vi "BeamGage Chart.vi"() -> ()   [LabVIEW 2009]
uses:
  C:/Program Files/Spiricon/BeamGage Professional/Spiricon.BeamGage.Automation.dll
  C:/Program Files/Spiricon/BeamGage Professional/Spiricon.Automation.dll
panel:
  out "Status":i32(ring) items=["NOT_SUPPORTED", "FAILED", "CALIBRATING", "READY", "BEAM_DETECTED"]
  out "2D Intensity Graph":dbl[][](graph)
  out "1D Profile - Peak Location Y - Waveform Graph":dbl[](graph)
  out "Height":dbl
  out "Width":dbl
  out "Peak Loc Y":dbl
  out "Peak Loc X":dbl
  in  "START_STOP":bool
  in  "ULTRACAL":bool
  out "Total and Peak Power - Waveform Chart":cluster{"Total":dbl, "Peak":dbl}(graph)
  in  "STOP SERVER":bool
  # "Block laser beam and \nclick Ultracal to calibrate"
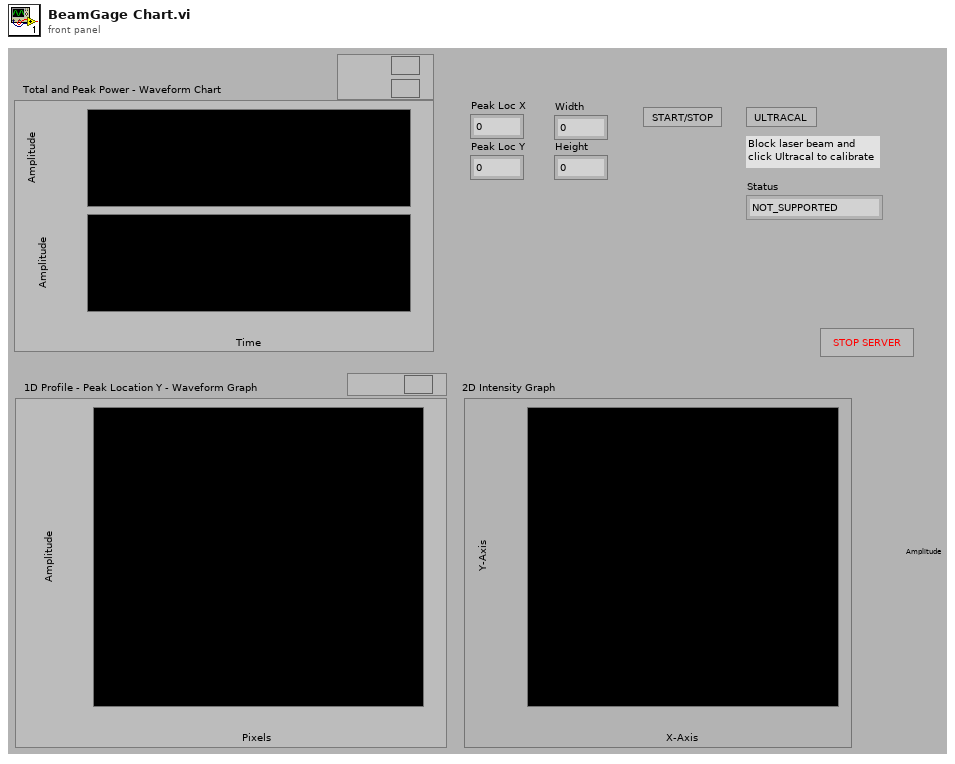
[diagram p1: front panel]
types:
  T1 = cluster{"Total":dbl, "Peak":dbl, "Peak X":dbl, "Peak Y":dbl, "Width":dbl, "Height":dbl, "DoubleData":dbl[], "Scale Multiplier":dbl}
  T2 = cluster{"notifier out":refnum<notifier>, "new reference":refnum<k24>}
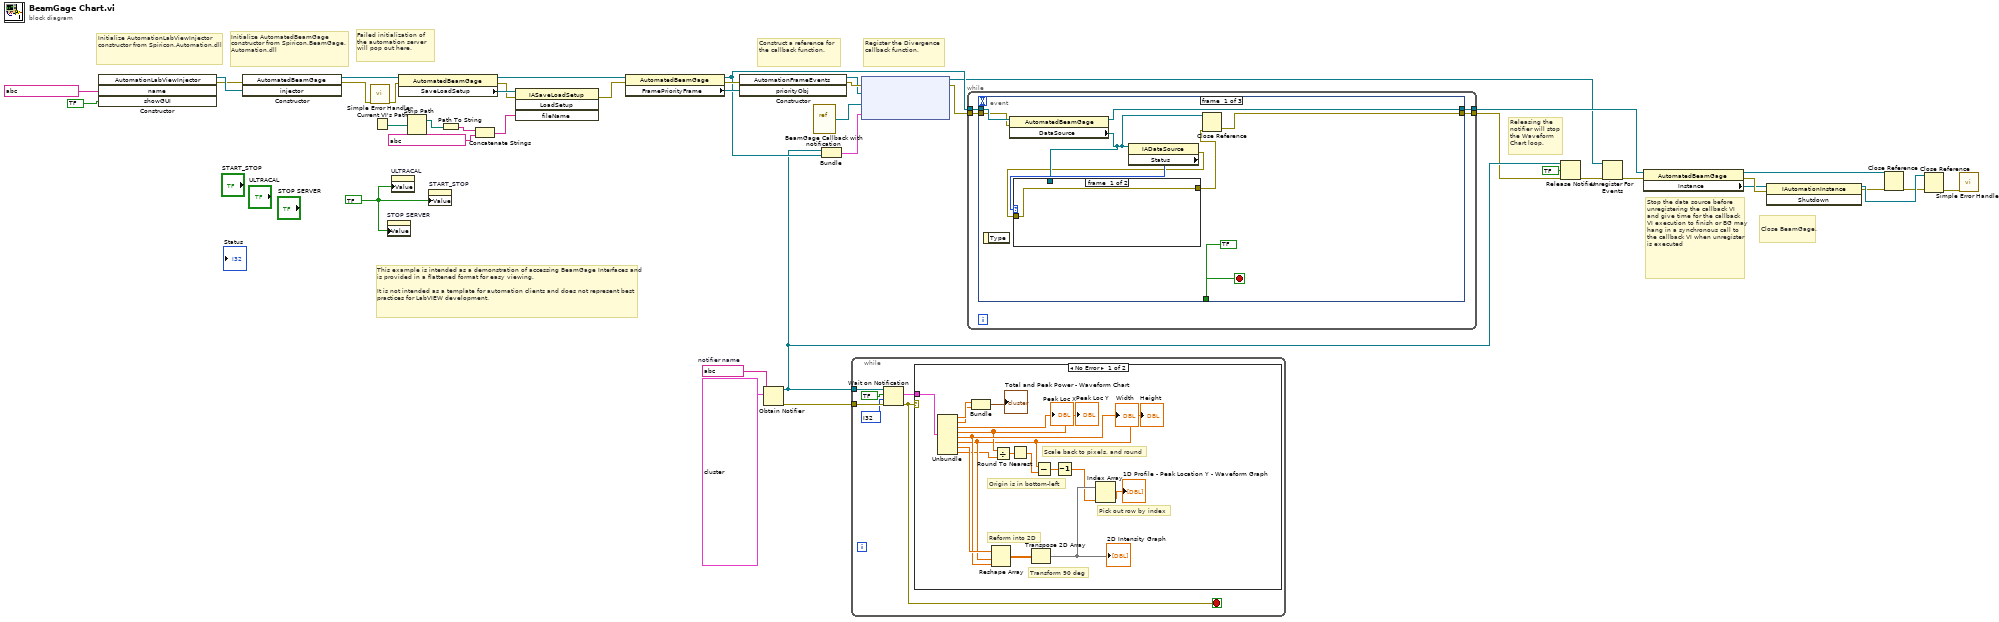
[diagram p0: block diagram]
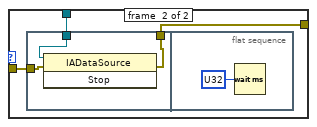
[diagram p2: hidden frame]
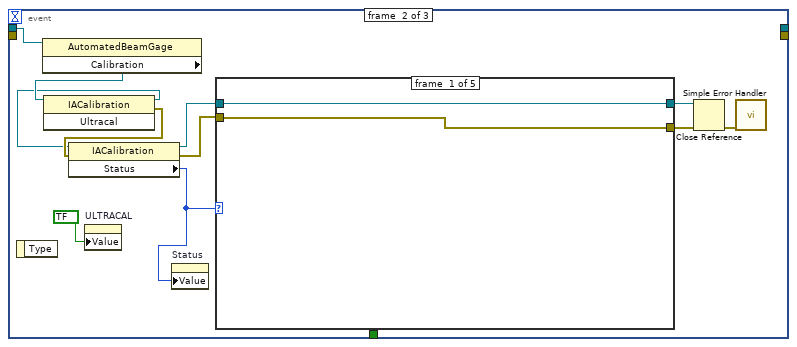
[diagram p3: hidden frame]
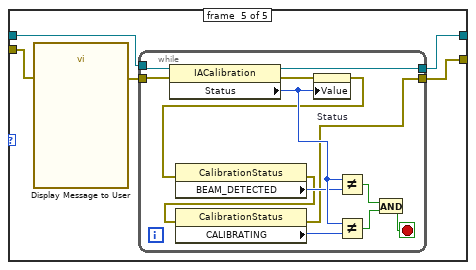
[diagram p7: hidden frame]
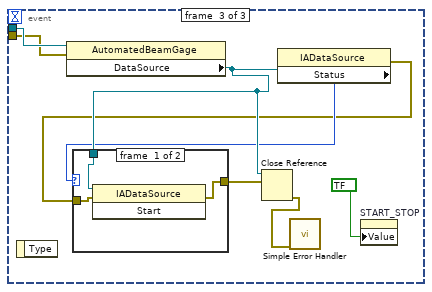
[diagram p8: hidden frame]
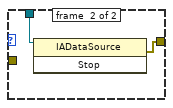
[diagram p9: hidden frame]
diagram:
  w39 = bool ? ("stop")
  w42 = string ?  # notifier name
  # "Initialize AutomationLabViewInjector constructor from Spiricon.Automation.dll"
  # "Failed initialization of the automation server will pop out here."
  # "This example is intended as a demonstration of accessing BeamGage Interfaces and is provided in a flattened format for easy viewing.\n\nIt is not intended as a template for automation clients and does not represent best practices for LabVIEW development."
  # "Stop the data source before unregistering the callback VI  and give time for the callback VI execution to finish or BG may hang in a synchronous call to the callback VI when unregister is executed"
  # "Releasing the notifier will stop the Waveform Chart loop."
  # "Close BeamGage."
  # "Initialize AutomatedBeamGage constructor from Spiricon.BeamGage.Automation.dll"
  # "Register the Divergence callback function."
  # "Construct a reference for the callback function."
  n1 = constructor class="AutomationLabViewInjector"("name"=string ? ("Name"), "showGUI"=bool ? ("LaunchUI")) -> (reference out=w4:refnum<k24>, error out=w1:errorcluster)  [unwired: 3 in, 3 out]
  n2 = constructor class="AutomatedBeamGage"(error in=w1, "injector"=w4) -> (reference out=w35:refnum<k24>, error out=w6:errorcluster)  [unwired: 2 in, 2 out]
  n3 = call <vilib>:"Simple Error Handler.vi"("error in (no error)"=w6) -> ("error out"=w5:errorcluster)  [unwired: 4 in, 4 out]
  n4 = Current VI's Path() -> (path=w28:path)
  n5 = property on="STOP SERVER" class="Bool (strict)"("Value"=w39) -> ()  [unwired: 2 in, 2 out]
  n6 = property on="ULTRACAL" class="Bool (strict)"("Value"=w39) -> ()  [unwired: 2 in, 2 out]
  n7 = property class="AutomatedBeamGage"(reference=w35, error in=w5) -> (reference out=w31:refnum<k24>, error out=w33:errorcluster, "SaveLoadSetup"=w34:refnum<k24>)
  n8 = Strip Path(path=w28) -> (stripped path=w27:path)  [unwired: 1 out]
  n9 = property on="START_STOP" class="Bool (strict)"("Value"=w39) -> ()  [unwired: 2 in, 2 out]
  n10 = Path To String(path=w27) -> (string=w30:string)
  n11 = Concatenate Strings(w30, string ? ("string")) -> (w26:string)
  n12 = invoke class="IASaveLoadSetup" method="LoadSetup"(reference=w34, error in=w33, "fileName"=w26) -> (error out=w32:errorcluster)  [unwired: 1 in, 3 out]
  n13 = property class="AutomatedBeamGage"(reference=w31, error in=w32) -> (reference out=w36:refnum<k24>, error out=w37:errorcluster, "FramePriorityFrame"=w38:refnum<k24>)
  n14 = constructor class="AutomationFrameEvents"(error in=w37, "priorityObj"=w38) -> (reference out=w24:refnum<k24>, error out=w25:errorcluster)  [unwired: 2 in, 2 out]
  n15 = Obtain Notifier(name (unnamed)=w42, notification data type=T1 ?) -> (notifier out=w9:refnum<notifier>, error out=w40:errorcluster)  [unwired: 2 in, 1 out]
  n16 = vi-ref "BeamGage Callback with notification.vi"() -> ("vi reference"=w21:refnum<vi>)
  n17 = Bundle("notifier out"=w9, "new reference"=w36) -> (w22:T2)  [unwired: 1 in]
  n18 = while {
    tunnel: w9 -> [w48]
    tunnel: w40 -> [w46]
    stop <- w44 stop-if-true
    n19 = Wait on Notification(notifier=w48, ignore previous (F)=bool ?, timeout in ms (-1)=i32 ?, error in (no error)=w46) -> (notification=w47:T1, error out=w44:errorcluster)  [unwired: 2 out]
    n20 = case shown="No Error" w44 {
      tunnel: w47 -> [w65 _]
      frame #0 {
        # "Transform 90 deg"
        # "Scale back to pixels, and round"
        # "Pick out row by index"
        # "Reform into 2D"
        # "Origin is in bottom-left"
        n21 = Unbundle(w65) -> ("Total"=w64:dbl, "Peak"=w63:dbl, "Peak X"=→"Peak Loc X":dbl, "Peak Y"=w54:dbl, "Width"=w56:dbl, "Height"=w52:dbl, "DoubleData"=w59:dbl[], "Scale Multiplier"=w49:dbl)
        "Peak Loc Y" <- w54
        "Width" <- w56
        "Height" <- w52
        n22 = Bundle("Total"=w64, "Peak"=w63) -> (→"Total and Peak Power - Waveform Chart":cluster{"Total":dbl, "Peak":dbl})  [unwired: 1 in]
        n23 = Reshape Array(w59, w52, w56) -> (w58:dbl[][])
        n24 = Divide(x=w54, y=w49) -> (x/y=w55:dbl)
        n25 = Round To Nearest(number=w55) -> (nearest integer value=w51:dbl)
        n26 = Transpose 2D Array(2D array=w58) -> (transposed array=w57:dbl[][])
        "2D Intensity Graph" <- w57
        n27 = Subtract(x=w52, y=w51) -> (x-y=w53:dbl)
        n28 = Decrement(x=w53) -> (x-1=w50:dbl)
        n29 = Index Array(array=w57, index (col)=w50) -> (element=→"1D Profile - Peak Location Y - Waveform Graph":dbl[])  [unwired: 1 in]
      }
      frame #1 {
        # "Don't update chart when an error occurs."
      }
    }
  }
  n30 = node(w25, w24, w21, w22) -> (w10:refnum<k27>, w23:errorcluster)  [unwired: 1 in]
  n31 = while {
    tunnel: [w70] -> w11
    tunnel: w36 -> [w69]
    tunnel: w23 -> [w67]
    tunnel: [w66] -> w8
    stop <- w68 stop-if-true
    n32 = event shown="[1] \"ULTRACAL\": Mouse Down" {
      selector: _ -> [_ _ _]
      dyn-events: _ -> [_ _ _]
      timeout: _ -> [_ _ _]
      tunnel: w69 -> [w77 w97 w129]
      tunnel: [w76 _ _] -> w70
      tunnel: [bool ? ("stop") _ _] -> w68
      tunnel: w67 -> [w75 _ w128]
      tunnel: [w78 _ _] -> w66
      event #0 {
        n33 = event-data() -> ()  [unwired: 1 in, 1 out]
        n34 = property class="AutomatedBeamGage"(reference=w77, error in=w75) -> (reference out=w76:refnum<k24>, "DataSource"=w73:refnum<k24>)  [unwired: 1 out]
        n35 = property class="IADataSource"(reference=w73) -> (error out=w71:errorcluster, "Status"=w74:i32)  [unwired: 1 in, 1 out]
        n36 = case shown="1" w74 {
          tunnel: w73 -> [_ w83]
          tunnel: [w80 w82] -> w72
          tunnel: w71 -> [w80 w81]
          frame #0 {
          }
          frame #1 {
            n37 = flat-sequence {
              tunnel: w83 -> [w86]
              tunnel: [w85] -> w82
              tunnel: w81 -> [w84]
              frame #0 {
                n38 = invoke class="IADataSource" method="Stop"(reference=w86, error in=w84) -> (error out=w85:errorcluster)  [unwired: 1 in, 2 out]
              }
              frame #1 {
                n39 = Wait (ms)(milliseconds to wait=u32 ?) -> ()  [unwired: 1 out]
              }
            }
          }
        }
        n40 = Close Reference(reference=w73, error in (no error)=w72) -> (error out=w78:errorcluster)
      }
      event #1 {
        n41 = event-data() -> ()  [unwired: 1 in, 1 out]
        n42 = property class="AutomatedBeamGage"(reference=w97) -> ("Calibration"=w96:refnum<k24>)  [unwired: 1 in, 2 out]
        n43 = invoke class="IACalibration" method="Ultracal"(reference=w96) -> (reference out=w94:refnum<k24>, error out=w95:errorcluster)  [unwired: 2 in, 1 out]
        n44 = property class="IACalibration"(reference=w94, error in=w95) -> (reference out=w93:refnum<k24>, error out=w92:errorcluster, "Status"=w91:i32)
        n45 = property on="ULTRACAL" class="Bool (strict)"("Value"=bool ? ("stop")) -> ()  [unwired: 2 in, 2 out]
        n46 = property on="Status" class="Ring (strict)"("Value"=w91) -> ()  [unwired: 2 in, 2 out]
        n47 = case shown="4" w91 {
          tunnel: [w99 w101 w103 w105 w107] -> w88
          tunnel: [w100 w102 w104 w106 w109] -> w89
          tunnel: w93 -> [w100 w102 w104 w106 w110]
          tunnel: w92 -> [w99 w101 w103 w105 w111]
          frame #0 {
          }
          frame #1 {
          }
          frame #2 {
          }
          frame #3 {
          }
          frame #4 {
            n48 = call "Display Message to User"("error in (no error)"=w111) -> ("error out"=w108:errorcluster)  [unwired: 9 in, 1 out]
            n49 = while {
              tunnel: w110 -> [w124]
              tunnel: [w123] -> w109
              tunnel: w108 -> [w122]
              tunnel: [w112] -> w107
              stop <- w120 stop-if-true
              n50 = property class="IACalibration"(reference=w124, error in=w122) -> (reference out=w123:refnum<k24>, error out=w121:errorcluster, "Status"=w117:i32)
              n51 = property on="Status" class="Ring (strict)"(error in=w121, "Value"=w117) -> (error out=w116:errorcluster)  [unwired: 1 in, 1 out]
              n52 = property class="CalibrationStatus"(error in=w116) -> (error out=w113:errorcluster, "BEAM_DETECTED"=w115:i32)  [unwired: 1 in, 1 out]
              n53 = property class="CalibrationStatus"(error in=w113) -> (error out=w112:errorcluster, "CALIBRATING"=w114:i32)  [unwired: 1 in, 1 out]
              n54 = Not Equal?(x=w117, y=w115) -> (x != y?=w118:bool)
              n55 = Not Equal?(x=w117, y=w114) -> (x != y?=w119:bool)
              n56 = And(x=w118, y=w119) -> (x .and. y?=w120:bool)
            }
          }
        }
        n57 = Close Reference(reference=w89, error in (no error)=w88) -> (error out=w90:errorcluster)
        n58 = call <vilib>:"Simple Error Handler.vi"("error in (no error)"=w90) -> ()  [unwired: 4 in, 5 out]
      }
      event #2 {
        n59 = event-data() -> ()  [unwired: 1 in, 1 out]
        n60 = property class="AutomatedBeamGage"(reference=w129, error in=w128) -> ("DataSource"=w127:refnum<k24>)  [unwired: 2 out]
        n61 = property class="IADataSource"(reference=w127) -> (error out=w125:errorcluster, "Status"=w126:i32)  [unwired: 1 in, 1 out]
        n62 = case shown="1" w126 {
          tunnel: [w133 w137] -> w131
          tunnel: w127 -> [w135 w136]
          tunnel: w125 -> [w134 _]
          frame #0 {
            n63 = invoke class="IADataSource" method="Start"(reference=w135, error in=w134) -> (error out=w133:errorcluster)  [unwired: 1 in, 2 out]
          }
          frame #1 {
            n64 = invoke class="IADataSource" method="Stop"(reference=w136) -> (error out=w137:errorcluster)  [unwired: 2 in, 2 out]
          }
        }
        n65 = Close Reference(reference=w127, error in (no error)=w131) -> (error out=w130:errorcluster)
        n66 = call <vilib>:"Simple Error Handler.vi"("error in (no error)"=w130) -> ()  [unwired: 4 in, 5 out]
        n67 = property on="START_STOP" class="Bool (strict)"("Value"=bool ? ("stop")) -> ()  [unwired: 2 in, 2 out]
      }
    }
  }
  n68 = Release Notifier(notifier=w9, force destroy? (F)=bool ?, error in (no error)=w8) -> (error out=w12:errorcluster)  [unwired: 2 out]
  n69 = Unregister For Events(event registration refnum=w10, error in=w12) -> (error out=w16:errorcluster)
  n70 = property class="AutomatedBeamGage"(reference=w11, error in=w16) -> (reference out=w15:refnum<k24>, error out=w17:errorcluster, "Instance"=w14:refnum<k24>)
  n71 = invoke class="IAutomationInstance" method="Shutdown"(reference=w14, error in=w17) -> (reference out=w19:refnum<k24>, error out=w13:errorcluster)  [unwired: 1 in, 1 out]
  n72 = Close Reference(reference=w15, error in (no error)=w13) -> (error out=w18:errorcluster)
  n73 = Close Reference(reference=w19, error in (no error)=w18) -> (error out=w7:errorcluster)
  n74 = call <vilib>:"Simple Error Handler.vi"("error in (no error)"=w7) -> ()  [unwired: 4 in, 5 out]
